vi "DAQmx Reference Trigger (Digital Edge).vi"(0 "task/channels in":refnum<k21>, 5 "source":tag, 7 "edge":i32(ring)=10280 items=["Rising"=10280, "Falling"=10171], 11 "error in":errorcluster, 12 "pretrigger samples per channel":u32=500) -> (4 "task out":refnum<k21>, 15 "error out":errorcluster)   [LabVIEW 2011]
doc: "Configures the task to stop the acquisition when the device acquires all pretrigger samples, detects a rising or falling edge of a digital signal, and acquires all posttrigger samples. When you use a Reference Trigger, the default for the read RelativeTo property is <B>First Pretrigger Sample</B> with a read Offset of 0."
uses:
  C:/Program Files/National Instruments/LabVIEW 2011/resource/objmgr/daqmx.rc
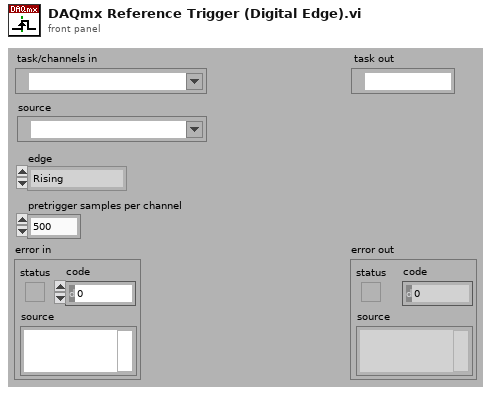
[diagram p1: front panel]
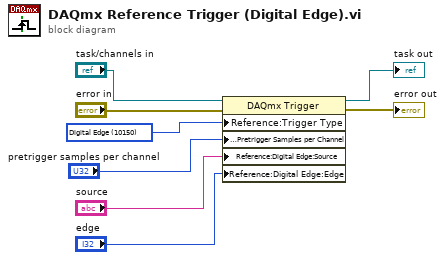
[diagram p0: block diagram]
diagram:
  w3 = 10150 items=["Analog Edge"=10099, "Digital Edge"=10150, "Analog Window"=10103, "None"=10230] ("Reference:Trigger Type")
  n1 = property class="DAQmx Trigger"(reference="task/channels in", error in="error in", "Reference:Trigger Type"=w3, "Reference:Pretrigger Samples per Channel"="pretrigger samples per channel", "Reference:Digital Edge:Source"="source", "Reference:Digital Edge:Edge"="edge") -> (reference out=→"task out":refnum<k21>, error out=→"error out":errorcluster)
